vi "Variant Attributes to JSON string.vi"(1 "Variant Attributes":variant) -> (0 "String":string)   [LabVIEW 2018]
uses:
  <vilib>/addons/_JKI.lib/Serialization/JSON/JKI JSON Serialization.lvlib
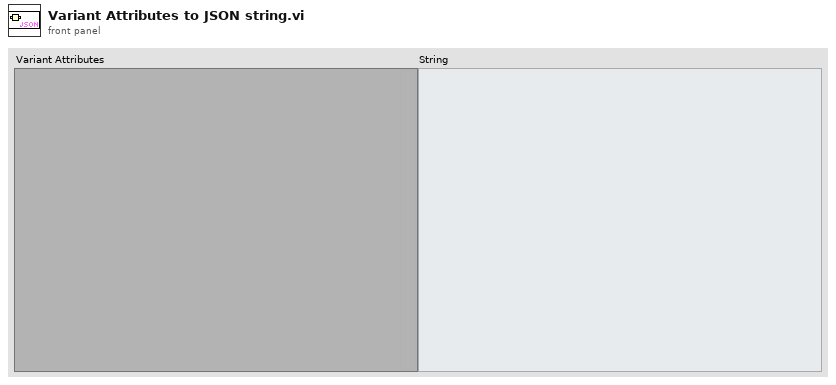
[diagram p1: front panel]
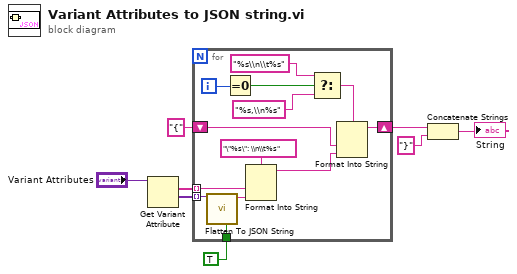
[diagram p0: block diagram]
diagram:
  n1 = Get Variant Attribute(Variant="Variant Attributes") -> (names=w3:string[], values=w4:variant[])  [unwired: 3 in, 2 out]
  n2 = for {
    tunnel: w3 -> [w19] mode=indexing
    tunnel: w4 -> [w21] mode=indexing
    shift-right: [w11] -> w6
    shift-left: "{" -> [w12]
    tunnel: TRUE ("Enums As String (F)") -> [w9]
    i -> [w14]
    n3 = call <vilib>:"Flatten To JSON String.vi"("Enums As String (F)"=w9, "Variant"=w21) -> ("JSON String"=w20:string)  [unwired: 8 in, 1 out]
    n4 = Equal To 0?(x=w14) -> (x = 0?=w17:bool)
    n5 = Format Into String(format string="\"%s\": \\n\\t%s", w19, w20) -> (resulting string=w10:string)  [unwired: 2 in, 1 out]
    n6 = Select(t="%s\\n\\t%s", s=w17, f="%s,\\n%s") -> (s? t:f=w13:string)
    n7 = Format Into String(format string=w13, w12, w10) -> (resulting string=w11:string)  [unwired: 2 in, 1 out]
  }
  n8 = Concatenate Strings(w6, "}" ("string")) -> (→"String":string)
